vi "ADC_pixis.vi"(6 "ADC offset":i32=-1 min=-1 step=1, 7 "ADC Gain":i32=-1 min=-1 step=1, 8 "error in (no error)":errorcluster, 9 "ADC Speed":i32=-1 min=-3 step=1, 10 "Read Out port":i32=-1 min=-1 step=1, 11 "Camera Handle":u32) -> (0 "error out":errorcluster, 1 "string":string, 2 "INI Flag":bool, 3 "Camera Handle":u32)   [LabVIEW 2015]
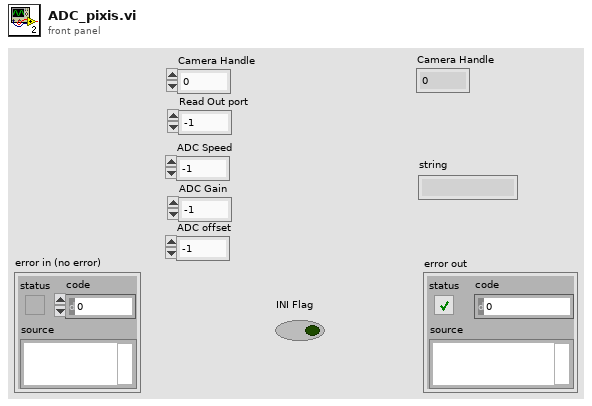
[diagram p1: front panel]
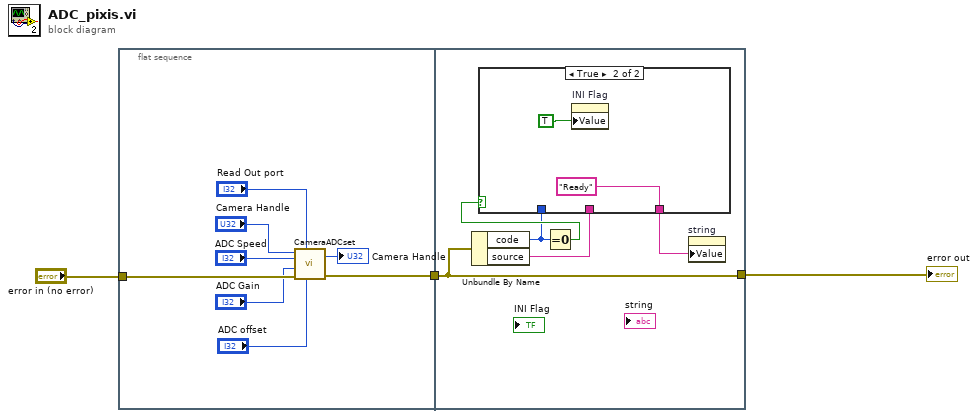
[diagram p0: block diagram]
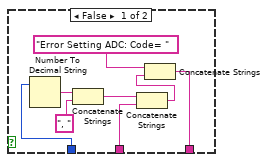
[diagram p2: hidden frame]
diagram:
  n1 = flat-sequence {
    tunnel: [w11] -> w2
    tunnel: "error in (no error)" -> [w10]
    tunnel: w2 -> [w13]
    tunnel: [w13] -> w1
    frame #0 {
      n2 = call <userlib>:"CameraADCset.vi"("ADC offset"="ADC offset", "Read Out port"="Read Out port", "error in (no error)"=w10, "ADC Gain"="ADC Gain", "ADC Speed"="ADC Speed", "Camera Handle"="Camera Handle") -> ("error out"=w11:errorcluster, "Camera Handle"=→"Camera Handle":u32)
    }
    frame #1 {
      n3 = Unbundle By Name(w13) -> ("code"=w14:i32, "source"=w15:string)
      n4 = Equal To 0?(x=w14) -> (x = 0?=w16:bool)
      n5 = case shown="True" w16 {
        tunnel: [w17 "Ready"] -> w12
        tunnel: w15 -> [w18 _]
        tunnel: w14 -> [w23 _]
        frame False {
          n6 = Number To Decimal String(number=w23) -> (decimal integer string=w22:string)  [unwired: 1 in]
          n7 = Concatenate Strings(w22, ", ") -> (w19:string)
          n8 = Concatenate Strings(w19, w18) -> (w20:string)
          n9 = Concatenate Strings("Error Setting ADC: Code= ", w20) -> (w17:string)
        }
        frame True {
          n10 = property on="INI Flag" class="Bool (strict)"("Value"=TRUE) -> ()  [unwired: 2 in, 2 out]
        }
      }
      n11 = property on="string" class="Str"("Value"=w12) -> ()  [unwired: 2 in, 2 out]
    }
  }
  "error out" <- w1
